vi "Remove Duplicates In Array.vi"(9 "Max Index Bound":i32, 11 "Random Numbers Array":i32[](array[numeric])) -> (3 "Random Numbers Array without Duplicates":i32[](array[numeric]))   [LabVIEW 2013]
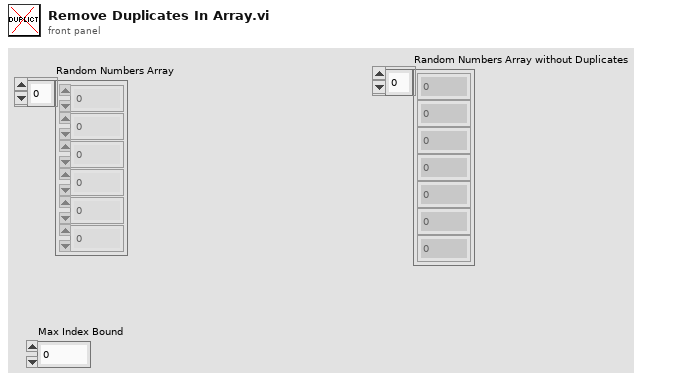
[diagram p1: front panel]
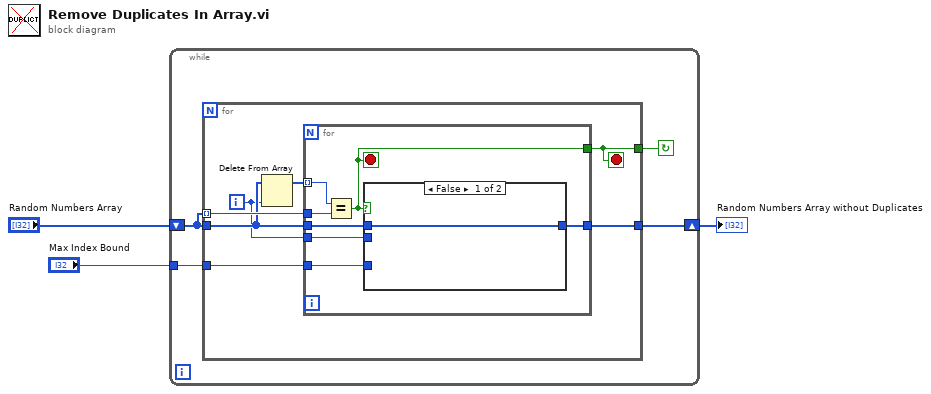
[diagram p0: block diagram]
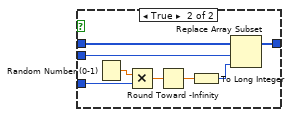
[diagram p2: hidden frame]
diagram:
  n1 = while {
    tunnel: "Max Index Bound" -> [w6]
    shift-right: [w4] -> w1
    shift-left: "Random Numbers Array" -> [w7]
    stop <- w5 continue-if-true
    n2 = for {
      tunnel: w7 -> [w13] mode=indexing
      tunnel: w7 -> [w11]
      tunnel: w6 -> [w12]
      tunnel: [w9] -> w4
      tunnel: [w8] -> w5
      i -> [w10]
      stop <- w8 stop-if-true
      n3 = Delete From Array(array=w11, index=w10) -> (array with subset deleted=w14:i32[])  [unwired: 1 in, 1 out]
      n4 = for {
        tunnel: w14 -> [w21] mode=indexing
        tunnel: w13 -> [w20]
        tunnel: w12 -> [w19]
        tunnel: w11 -> [w18]
        tunnel: w10 -> [w17]
        tunnel: [w16] -> w9
        tunnel: [w15] -> w8
        stop <- w15 stop-if-true
        n5 = Equal?(x=w21, y=w20) -> (x = y?=w15:bool)
        n6 = case shown="False" w15 {
          tunnel: w19 -> [_ w28]
          tunnel: w18 -> [w22 w27]
          tunnel: w17 -> [_ w24]
          tunnel: [w22 w23] -> w16
          frame False {
          }
          frame True {
            n7 = Random Number (0-1)() -> (number: 0 to 1=w30:dbl)
            n8 = Multiply(x=w30, y=w28) -> (x*y=w29:dbl)
            n9 = Round Toward -Infinity(1:w29) -> (0:w26:dbl)
            n10 = To Long Integer(number=w26) -> (32bit integer=w25:i32)
            n11 = Replace Array Subset(array=w27, new element=w25, index=w24) -> (w23:i32[])
          }
        }
      }
    }
  }
  "Random Numbers Array without Duplicates" <- w1
